vi "Change Actor Label.vi"(8 "error in (no error)":errorcluster, 10 "New Label":string, 11 "Recipe Window in":refnum<class "Recipe Window.lvclass">) -> (0 "error out":errorcluster, 3 "Recipe Window out":refnum<class "Recipe Window.lvclass">)   [LabVIEW 2021, in "Recipe.lvlib" / "Recipe Window.lvclass"]
uses:
  Recipe Window.lvclass
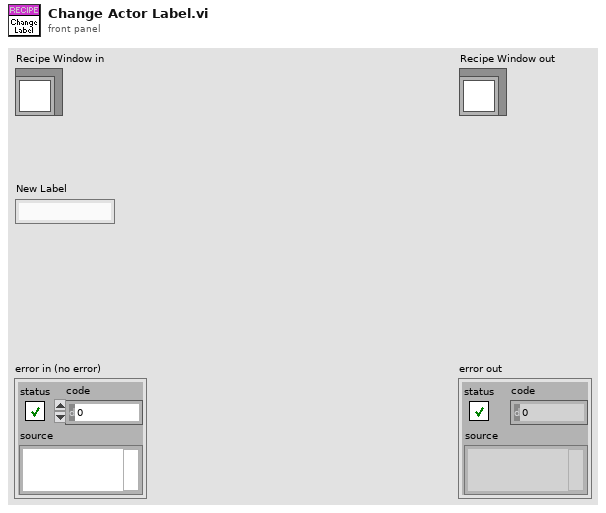
[diagram p1: front panel]
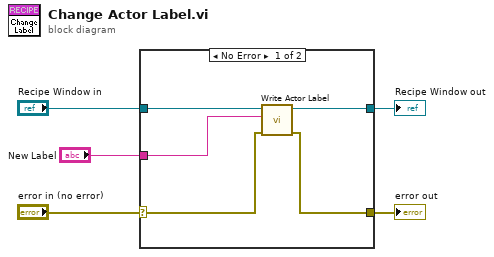
[diagram p0: block diagram]
diagram:
  n1 = case shown="No Error" "error in (no error)" {
    selector: "error in (no error)" -> [w7 w12]
    tunnel: [w6 w12] -> w4
    tunnel: [w10 w11] -> w1
    tunnel: "Recipe Window in" -> [w9 w11]
    tunnel: "New Label" -> [w8 _]
    frame No Error {
      n2 = call-dynamic "Write Actor Label.vi"("error in (no error)"=w7, "Actor Label"=w8, "Monitored Actor in"=w9) -> ("error out"=w6:errorcluster, "Monitored Actor out"=w10:refnum<class "Recipe Window.lvclass">)  [unwired: 7 in]
    }
    frame Error {
    }
  }
  "error out" <- w4
  "Recipe Window out" <- w1
